vi "Write error.vi"(0 "error in (no error)":errorcluster) -> ()   [LabVIEW 2013, in "AIT 664 Custom Device.lvlib"]
uses:
  AIT 664 Custom Device.lvlib
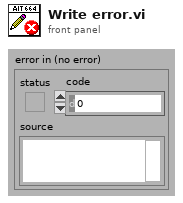
[diagram p1: front panel]
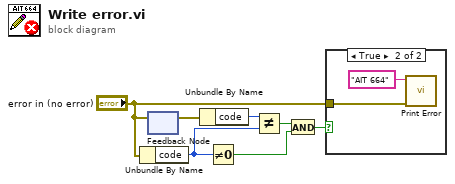
[diagram p0: block diagram]
diagram:
  n1 = Unbundle By Name("error in (no error)") -> ("code"=w3:i32)
  n2 = feedback #1() -> (w4:errorcluster)  [unwired: 1 in]
  n3 = feedback-in #1("error in (no error)") -> ()
  n4 = Unbundle By Name(w4) -> ("code"=w1:i32)
  n5 = Not Equal To 0?(x=w3) -> (x != 0?=w2:bool)
  n6 = Not Equal?(x=w1, y=w3) -> (x != y?=w6:bool)
  n7 = And(x=w6, y=w2) -> (x .and. y?=w5:bool)
  n8 = case shown="True" w5 {
    tunnel: "error in (no error)" -> [_ w9]
    frame False {
    }
    frame True {
      n9 = call "Print Error.vi"("error out"=w9, "Your code's public name"="AIT 664") -> ()  [unwired: 9 in]
    }
  }
